vi "Empty Host IO Resource.vi"() -> (0 "Host IO Resource":T1)   [LabVIEW 2021, in "Acquisition.lvlib"]
doc: "(inline VI) Return an empty Host IO Resource. Use in-place of a block diagram constant.\n\nA cluster representing an IO device discovered on the running Host system."
uses:
  Acquisition.lvlib
  Host IO Resource.ctl
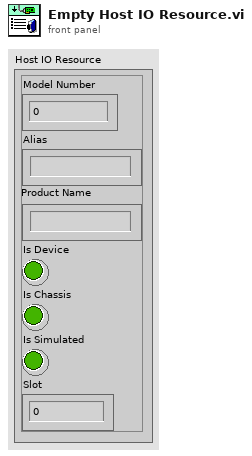
[diagram p1: front panel]
types:
  T1 = typedef "Acquisition.lvlib/Host IO Resource.ctl" = cluster{"Model Number":u32, "Alias":string, "Product Name":string, "Is Device":bool, "Is Chassis":bool, "Is Simulated":bool, "Slot":i32}
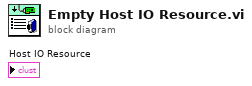
[diagram p0: block diagram]
diagram:
